vi "jtfa.vi"() -> ()   [LabVIEW 2023]
uses:
  <vilib>/Analysis/4window.llb/windowTd.ctl
  <vilib>/sound2/lvsound2.llb/Sampling Mode.ctl
  <vilib>/sound2/lvsound2.llb/Sound Data Format.ctl
  <vilib>/Analysis/2dsp.llb/Power Spectrum (DBL).vi
  <vilib>/Analysis/4window.llb/Hanning Window (DBL).vi
  <vilib>/Analysis/4window.llb/AllCosWindow (DBL).vi
  <vilib>/sound2/lvsound2.llb/Sound Input Read (DBL).vi
  <vilib>/addons/Time Frequency Analysis/_control.llb/TFA Configure Spectrogram Indicator (Predefined Color Table).vi
  <vilib>/Analysis/NI_AALPro.lvlib
  <vilib>/gmath/NI_Gmath.lvlib
  <vilib>/addons/_Advanced Signal Processing/NI_AdvSigProcTFA.lvlib
  <vilib>/express/express analysis/Spectral/XNode/ExpressSpectralMeasurementsBlockNode.xnode
  <vilib>/express/express analysis/Spectral/Block/exnSpectralBlock spectral measurements RMS poly.vi
  <vilib>/express/express analysis/Spectral/Block/exnSpectralBlock spectral measurements RMS DDT.vi
  <vilib>/Analysis/2dsp.llb/Real FFT.vi
  <vilib>/addons/Time Frequency Analysis/Spectrogram.llb/TFA Online STFT Spectrogram (Waveform).vi
  <vilib>/addons/Time Frequency Analysis/Spectrogram.llb/TFA STFT Spectrogram (Waveform).vi
  <vilib>/addons/Time Frequency Analysis/Transform.llb/TFA STFT (Waveform).vi
panel:
  in  "Num Samples/Ch (N)":dbl(slide)=4096.0 min=1.0 max=48000.0 scale=1.0..4096.0
  in  "Sample Time (s)":dbl(slide)=0.08533333333333333 min=0.01 max=2.0 scale=0.0..2.0
  in  "Frequency Resolution, df (Hz)":dbl(slide)=11.71875 min=1.0 max=24000.0 scale=1.0..100.0
  out "Spectrogram":dbl[][](graph)
  out "phase":dynamicdata(graph)
  out "waveform 2":dynamicdata(graph)
  out "spectrum 2":dynamicdata(graph)
  out "STFT":dbl[][](graph)
  in  "window info":cluster{"type":T1, "length":i32}={"type"=1, "length"=64} {"type" items=["Rectangle"=0, "Hanning"=1, "Hamming"=2, "Blackman-Harris"=3, "Exact Blackman"=4, "Blackman"=5, "Flat Top"=6, "4 Term B-Harris "=7, "7 Term B-Harris"=8, "Low Sidelobe"=9, "Blackman Nuttall"=11, "Triangle"=30, "Bartlett-Hanning"=31, "Bohman"=32, "Parzen"=33, "Welch"=34, "Kaiser"=60, "Dolph-Chebyshev"=61, "Gaussian"=62]}
  in  "time-freq sampling info":cluster{"time steps":i32, "frequency bins":i32}={"time steps"=-1, "frequency bins"=512}
  in  "hanning window":bool
  out "Nyquist Frequency (Hz)":dbl
  in  "stop":bool
  out "waveform":waveform(dbl)(graph)
  out "spectrum":waveform(dbl)(graph)
  # "left off 3am thu 4/11: persisted and got the code to work without errors, added bounds on the inputs to avoid errors (now only if go too low on T manually)\nnext: revisit assignment and what need to get done for that, look at chris sample code"
  # "!! want longer sampling window to get better freq resolution (?)\nb/c freq. res. = 1/time"
  # "w express vi"
  # "- can improve resolution by:\n-- increase length of fft window (but does make time res worse)\n-- increase num bins (increase freq res)"
  # "cut off at -100 dB (y)\ntrim x axis (auto goes\nout to nyq), but only go\nto 15000\n- turn off auto scaling"
  # "not sure why this isn't working but oh well just use chris' in morning"
  # "- our instrument\n- diff notes\n- compare to professional online"
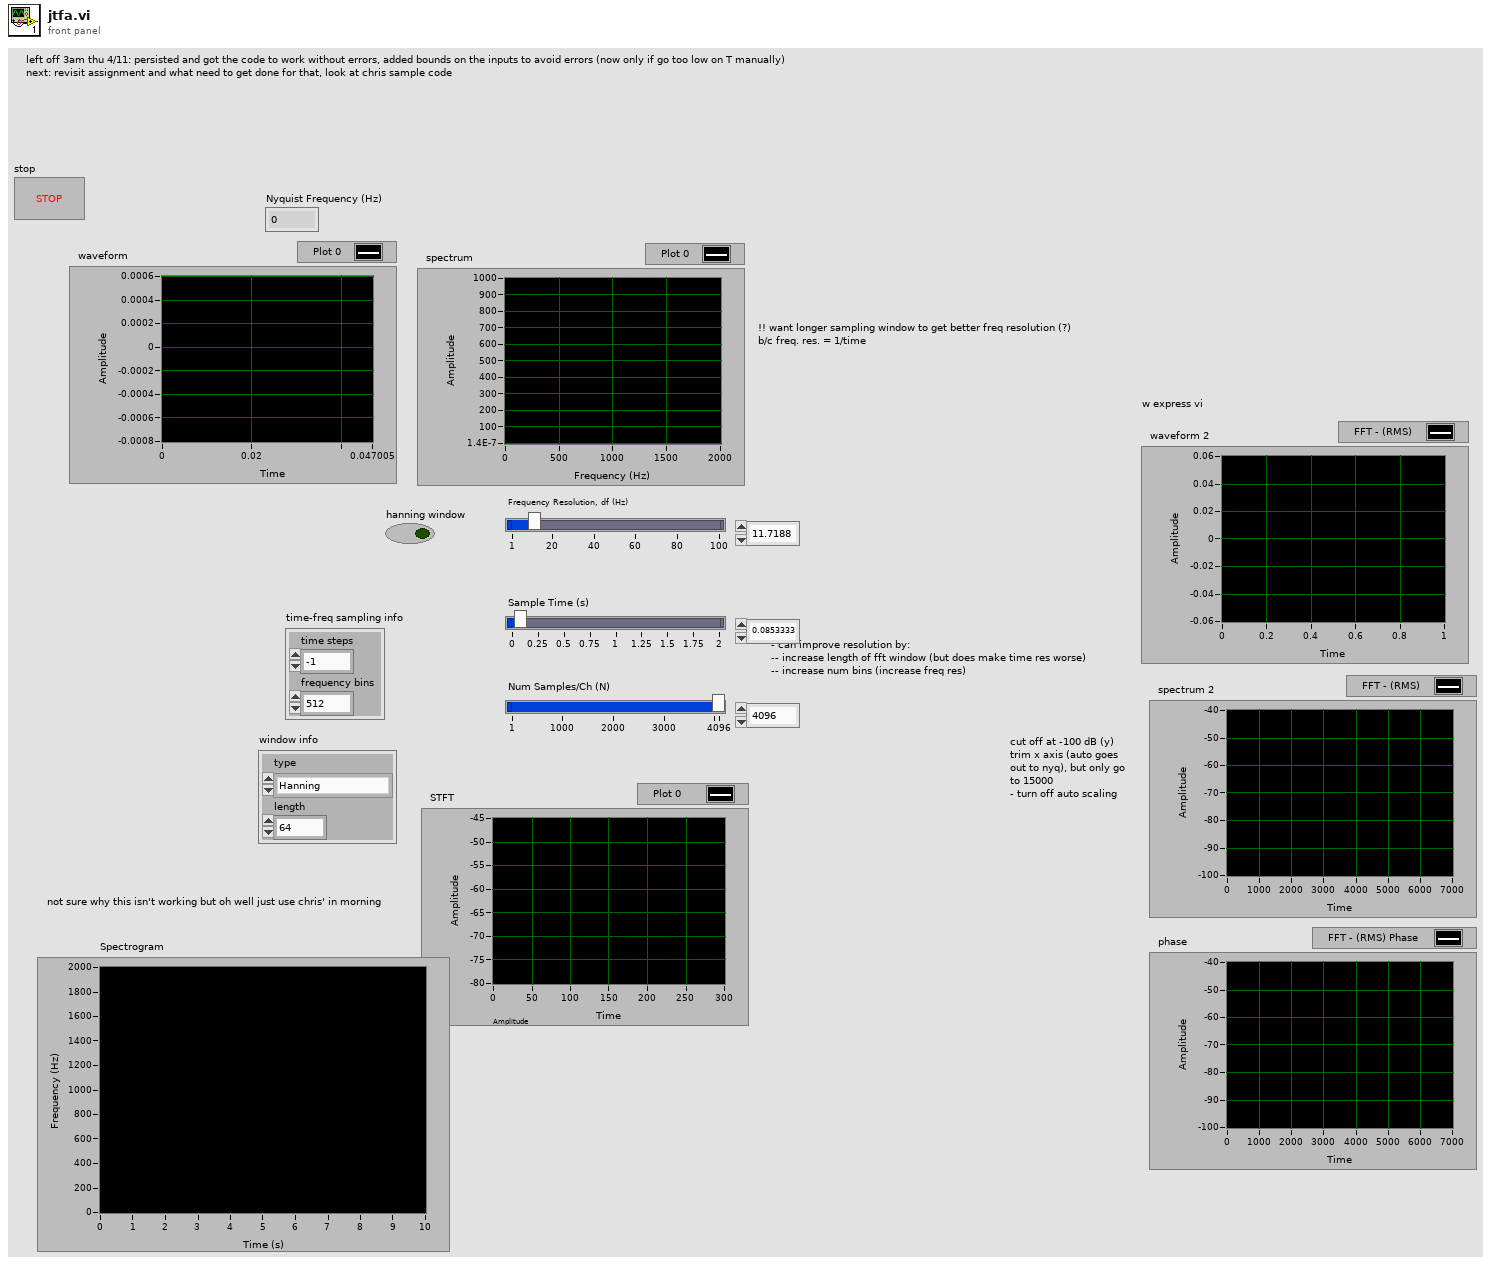
[diagram p1: front panel]
types:
  T1 = typedef "NI_AALPro.lvlib/windowTd.ctl" = u32
  T2 = typedef "Sound Data Format.ctl" = cluster{"sample rate (S/s)":dbl, "number of channels":i32, "bits per sample":i32}
  T3 = typedef "Sampling Mode.ctl" = i32
  T4 = typedef "Sound Input Task ID.ctl" = u32
  T5 = cluster{"averaging mode":u16, "weighting mode":u16, "number of averages":u32}
  T6 = cluster{"dB On (F)":bool, "unwrap phase (F)":bool, "convert to degree (F)":bool}
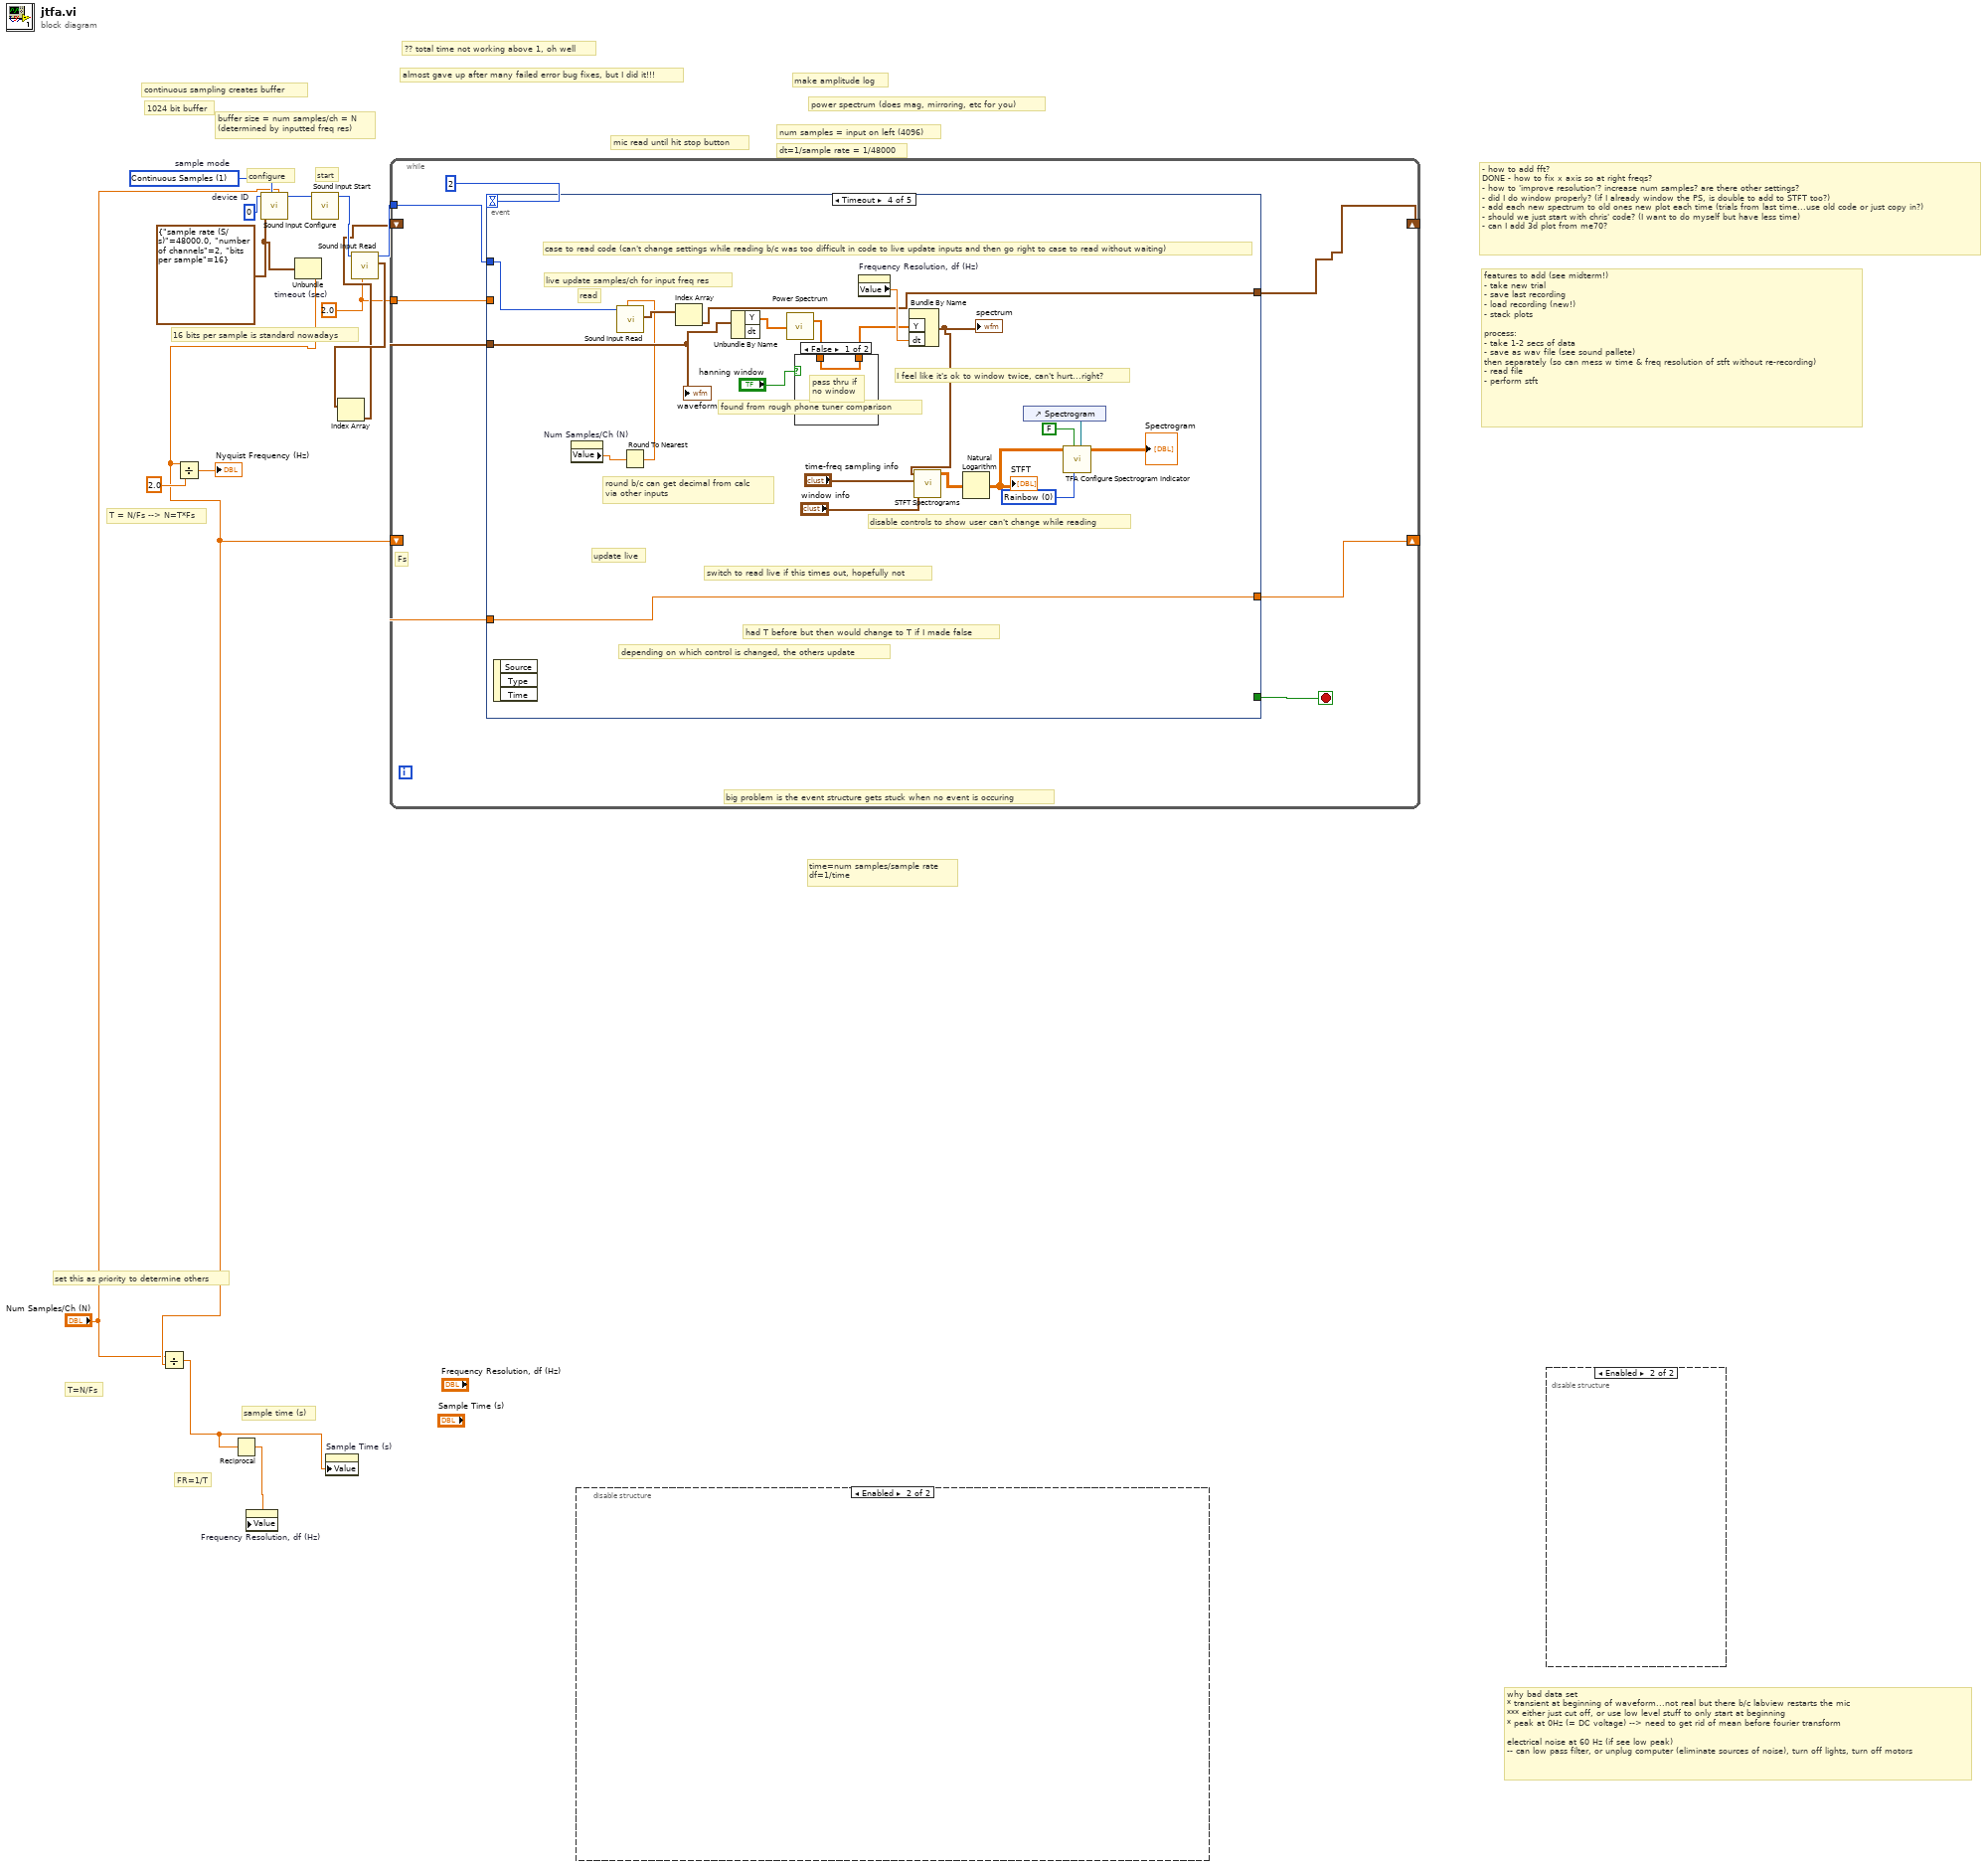
[diagram p0: block diagram]
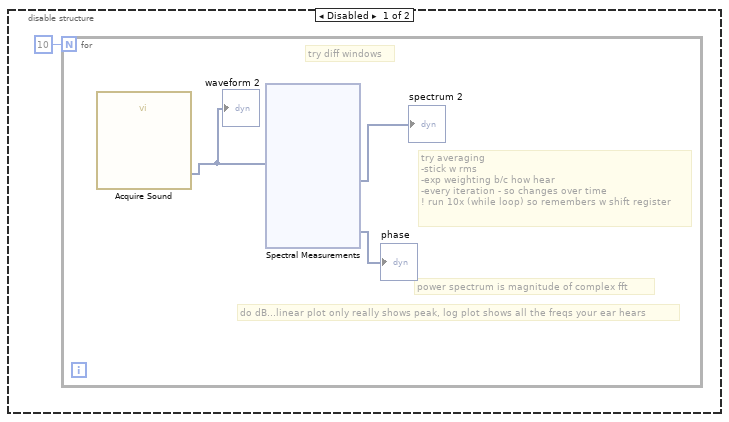
[diagram p2: hidden frame]
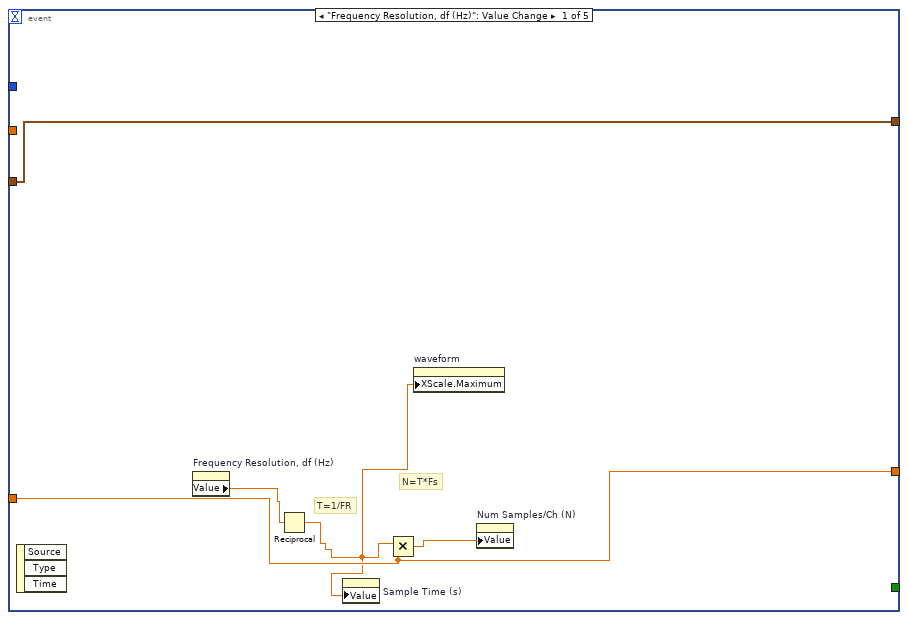
[diagram p3: hidden frame]
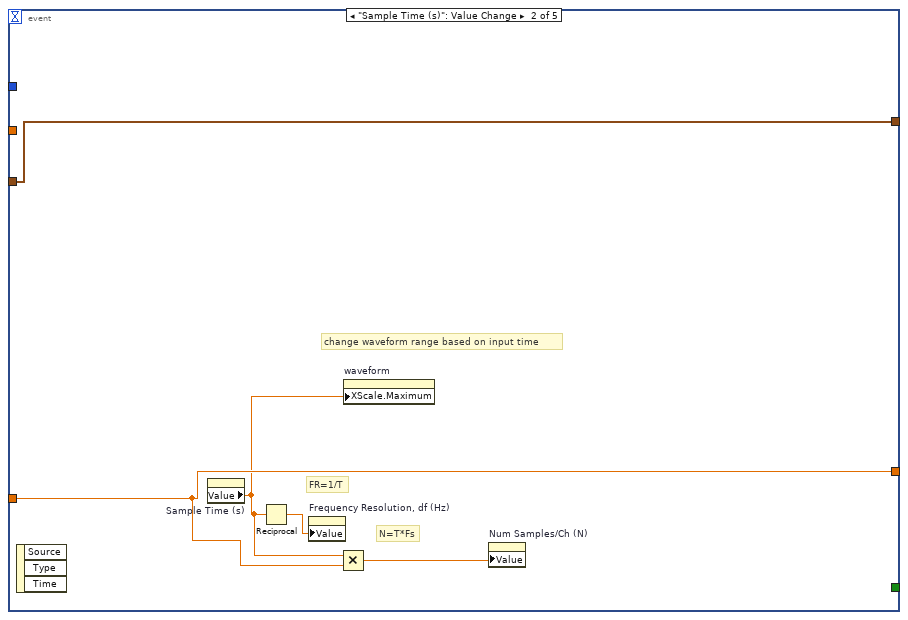
[diagram p4: hidden frame]
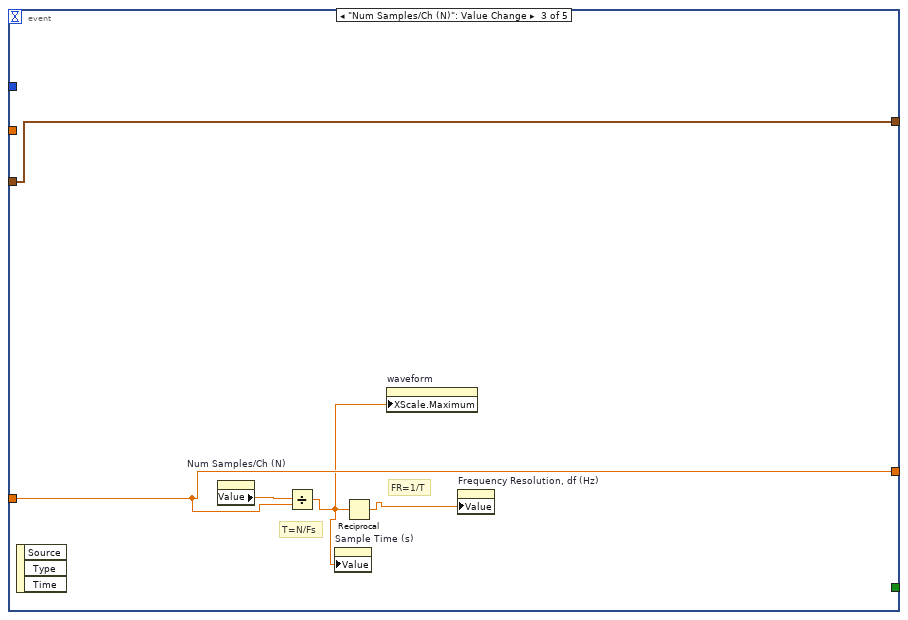
[diagram p5: hidden frame]
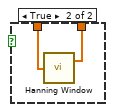
[diagram p6: hidden frame]
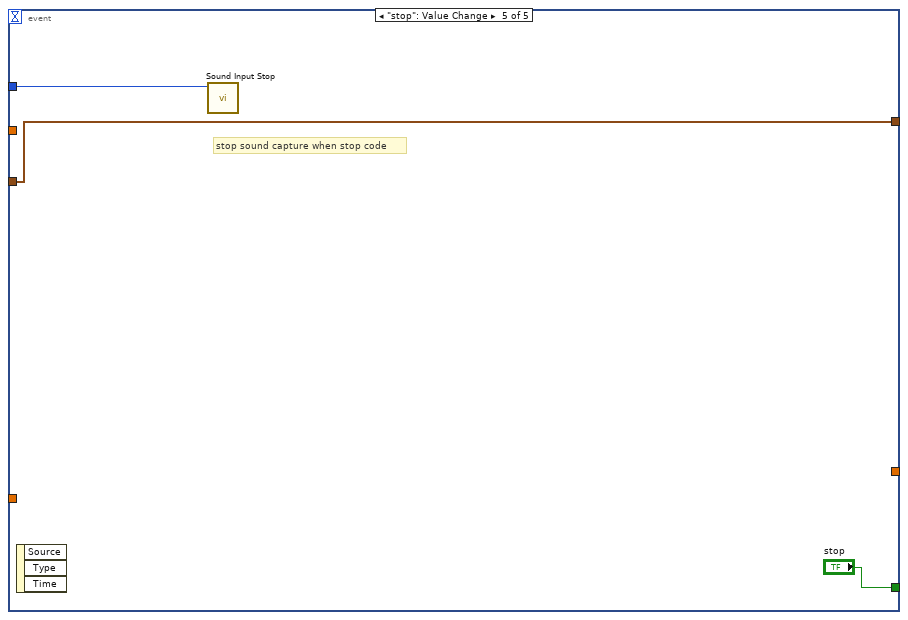
[diagram p7: hidden frame]
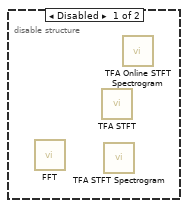
[diagram p8: hidden frame]
diagram:
  w5 = 2.0  # timeout (sec)
  w10 = T2 {"sample rate (S/s)"=48000.0, "number of channels"=2, "bits per sample"=16} ("sound format")
  w14 = u32 0  # device ID
  w15 = T3 1 items=["Finite Samples", "Continuous Samples"]  # sample mode
  # "?? total time not working above 1, oh well"
  # "almost gave up after many failed error bug fixes, but I did it!!!"
  # "FR=1/T"
  # "set this as priority to determine others"
  # "T=N/Fs"
  # "sample time (s)"
  # "T = N/Fs --> N=T*Fs"
  # "time=num samples/sample rate\ndf=1/time"
  # "num samples = input on left (4096)"
  # "dt=1/sample rate = 1/48000"
  # "buffer size = num samples/ch = N\n(determined by inputted freq res)"
  # "start"
  # "configure"
  # "make amplitude log"
  # "power spectrum (does mag, mirroring, etc for you)"
  # "16 bits per sample is standard nowadays"
  # "1024 bit buffer"
  # "continuous sampling creates buffer"
  # "mic read until hit stop button"
  # "why bad data set\n* transient at beginning of waveform...not real but there b/c labview restarts the mic\n*** either just cut off, or use low level stuff to only start at beginning\n* peak at 0Hz (= DC voltage) --> need to get rid of mean before fourier transform\n\nelectrical noise at 60 Hz (if see low peak)\n-- can low pass filter, or unplug computer (eliminate sources of noise), turn off lights, turn off motors"
  # "features to add (see midterm!)\n- take new trial\n- save last recording\n- load recording (new!)\n- stack plots\n\nprocess:\n- take 1-2 secs of data\n- save as wav file (see sound pallete)\nthen separately (so can mess w time & freq resolution of stft without re-recording)\n- read file\n- perform stft"
  # "- how to add fft?\nDONE - how to fix x axis so at right freqs?\n- how to 'improve resolution'? increase num samples? are there other settings?\n- did I do window properly? (if I already window the PS, is double to add to STFT too?)\n- add each new spectrum to old ones new plot each time (trials from last time...use old code or just copy in?)\n- should we just start with chris' code? (I want to do myself but have less time)\n- can I add 3d plot from me70?"
  n1 = call <vilib>:"Sound Input Configure.vi"("number of samples/ch"="Num Samples/Ch (N)", "sample mode"=w15, "sound format"=w10, "device ID"=w14) -> ("task ID"=w13:T4)  [unwired: 6 in, 1 out]
  n2 = Unbundle(w10) -> ("sample rate (S/s)"=w4:dbl)  [unwired: 2 out]
  n3 = Divide(x="Num Samples/Ch (N)", y=w4) -> (x/y=w2:dbl)
  n4 = Divide(x=w4, y=2.0) -> (x/y=→"Nyquist Frequency (Hz)":dbl)
  n5 = Reciprocal(x=w2) -> (1/x=w1:dbl)
  n6 = property on="Frequency Resolution, df (Hz)" class="Slide (strict)"("Value"=w1) -> ()  [unwired: 2 in, 2 out]
  n7 = call <vilib>:"Sound Input Start.vi"("task ID"=w13) -> ("task ID out"=w9:T4)  [unwired: 9 in, 1 out]
  n8 = property on="Sample Time (s)" class="Slide (strict)"("Value"=w2) -> ()  [unwired: 2 in, 2 out]
  n9 = call-poly <vilib>:"Sound Input Read.vi"("timeout (sec)"=w5, "task ID"=w9) -> ("data"=w7:waveform(dbl)[], "task ID out"=w8:T4)  [unwired: 7 in, 1 out]
  n10 = Index Array "Index Array"(array=w7) -> (element=w6:waveform(dbl))  [unwired: 1 in]
  n11 = while {
    shift-right: [w22] -> _
    shift-left: w4 -> [w23]
    tunnel: w8 -> [w20]
    shift-right: [w18] -> _
    shift-left: w6 -> [w17]
    tunnel: w5 -> [w16]
    stop <- w19 stop-if-true
    # "big problem is the event structure gets stuck when no event is occuring"
    # "Fs"
    n12 = event shown="[3] Timeout" {
      selector: _ -> [_ _ _ _ _]
      dyn-events: _ -> [_ _ _ _ _]
      timeout: 2 -> [_ _ _ _ _]
      tunnel: w23 -> [w26 w31 w36 w59 _]
      tunnel: [w26 w31 w36 w59 _] -> w22
      tunnel: w20 -> [_ _ _ w48 w65]
      tunnel: [_ _ _ _ "stop"] -> w19
      tunnel: [w25 w30 w35 w47 w63] -> w18
      tunnel: w17 -> [w25 w30 w35 w46 w63]
      tunnel: w16 -> [_ _ _ _ _]
      event "Frequency Resolution, df (Hz)": Value Change {
        # "N=T*Fs"
        # "T=1/FR"
        n13 = event-data() -> ()  [unwired: 1 in, 3 out]
        n14 = property on="Frequency Resolution, df (Hz)" class="Slide (strict)"() -> ("Value"=w28:dbl)  [unwired: 2 in, 2 out]
        n15 = Reciprocal(x=w28) -> (1/x=w24:dbl)
        n16 = property on="Sample Time (s)" class="Slide (strict)"("Value"=w24) -> ()  [unwired: 2 in, 2 out]
        n17 = Multiply(x=w24, y=w26) -> (x*y=w27:dbl)
        n18 = property on="waveform" class="WFGraph (strict)"("XScale.Maximum"=w24) -> ()  [unwired: 2 in, 2 out]
        n19 = property on="Num Samples/Ch (N)" class="Slide (strict)"("Value"=w27) -> ()  [unwired: 2 in, 2 out]
      }
      event "Sample Time (s)": Value Change {
        # "change waveform range based on input time"
        # "N=T*Fs"
        # "FR=1/T"
        n20 = event-data() -> ()  [unwired: 1 in, 3 out]
        n21 = property on="Sample Time (s)" class="Slide (strict)"() -> ("Value"=w29:dbl)  [unwired: 2 in, 2 out]
        n22 = Reciprocal(x=w29) -> (1/x=w33:dbl)
        n23 = property on="Frequency Resolution, df (Hz)" class="Slide (strict)"("Value"=w33) -> ()  [unwired: 2 in, 2 out]
        n24 = Multiply(x=w29, y=w31) -> (x*y=w32:dbl)
        n25 = property on="waveform" class="WFGraph (strict)"("XScale.Maximum"=w29) -> ()  [unwired: 2 in, 2 out]
        n26 = property on="Num Samples/Ch (N)" class="Slide (strict)"("Value"=w32) -> ()  [unwired: 2 in, 2 out]
      }
      event "Num Samples/Ch (N)": Value Change {
        # "T=N/Fs"
        # "FR=1/T"
        n27 = event-data() -> ()  [unwired: 1 in, 3 out]
        n28 = property on="Num Samples/Ch (N)" class="Slide (strict)"() -> ("Value"=w38:dbl)  [unwired: 2 in, 2 out]
        n29 = Divide(x=w38, y=w36) -> (x/y=w34:dbl)
        n30 = property on="Sample Time (s)" class="Slide (strict)"("Value"=w34) -> ()  [unwired: 2 in, 2 out]
        n31 = Reciprocal(x=w34) -> (1/x=w37:dbl)
        n32 = property on="waveform" class="WFGraph (strict)"("XScale.Maximum"=w34) -> ()  [unwired: 2 in, 2 out]
        n33 = property on="Frequency Resolution, df (Hz)" class="Slide (strict)"("Value"=w37) -> ()  [unwired: 2 in, 2 out]
      }
      event Timeout {
        w40 = u16 0 items=["Rainbow", "Inverse gray", "Gray"] ("color table")
        # "round b/c can get decimal from calc\nvia other inputs"
        # "disable controls to show user can't change while reading"
        # "case to read code (can't change settings while reading b/c was too difficult in code to live update inputs and then go right to case to read without waiting)"
        # "depending on which control is changed, the others update"
        # "live update samples/ch for input freq res"
        # "update live"
        # "I feel like it's ok to window twice, can't hurt...right?"
        # "found from rough phone tuner comparison"
        # "read"
        # "had T before but then would change to T if I made false"
        # "switch to read live if this times out, hopefully not"
        n34 = event-data() -> ()  [unwired: 1 in, 3 out]
        n35 = property on="Num Samples/Ch (N)" class="Slide (strict)"() -> ("Value"=w45:dbl)  [unwired: 2 in, 2 out]
        n36 = Round To Nearest(number=w45) -> (nearest integer value=w44:dbl)
        n37 = call-poly <vilib>:"Sound Input Read.vi"("number of samples/ch"=w44, "task ID"=w48) -> ("data"=w57:waveform(dbl)[])  [unwired: 7 in, 2 out]
        n38 = Index Array "Index Array"(array=w57) -> (element=w47:waveform(dbl))  [unwired: 1 in]
        n39 = Unbundle By Name(w46) -> ("Y"=w56:dbl[])  [unwired: 1 out]
        n40 = call-poly <vilib>:"Power Spectrum.vi"("X"=w56) -> ("Power Spectrum"=w54:dbl[])  [unwired: 1 out]
        n41 = case shown="False" "hanning window" {
          tunnel: w54 -> [w60 w62]
          tunnel: [w60 w61] -> w53
          frame False {
            # "pass thru if\nno window"
          }
          frame True {
            n42 = call-poly <vilib>:"Hanning Window.vi"("X"=w62) -> ("Windowed X"=w61:dbl[])  [unwired: 1 out]
          }
        }
        n43 = property on="Frequency Resolution, df (Hz)" class="Slide (strict)"() -> ("Value"=w58:dbl)  [unwired: 2 in, 2 out]
        n44 = Bundle By Name("Y"=w53, "dt"=w58) -> (w52:waveform(dbl))  [unwired: 1 in]
        "spectrum" <- w52
        n45 = call <vilib>:"STFT Spectrograms.vi"("window info"="window info", "time-freq sampling info"="time-freq sampling info", "X"=w52) -> ("STFT Spectrogram {X}"=w49:dbl[][])  [unwired: 7 in, 1 out]
        n46 = Natural Logarithm(1:w49) -> (0:w41:dbl[][])
        "STFT" <- w41
        n47 = control-ref of="Spectrogram"() -> (w42:refnum<vi>)
        n48 = call-poly <vilib>:"TFA Configure Spectrogram Indicator.vi"("reference of TF spectrogram indicator"=w42, "color table"=w40, "dB on? (F)"=FALSE, "spectrogram"=w41) -> ("TF spectrogram indicator"=→"Spectrogram":dbl[][])  [unwired: 3 in, 4 out]
        "waveform" <- w46
      }
      event "stop": Value Change {
        # "stop sound capture when stop code"
        n49 = event-data() -> ()  [unwired: 1 in, 3 out]
        n50 = call <vilib>:"Sound Input Stop.vi"("task ID"=w65) -> ()  [unwired: 9 in, 2 out]
      }
    }
  }
  n51 = disable-structure shown="Enabled" {
    frame Disabled {
      n52 = for {
        N: 10 -> [_]
        # "do dB...linear plot only really shows peak, log plot shows all the freqs your ear hears"
        # "try diff windows"
        # "power spectrum is magnitude of complex fft"
        # "try averaging\n-stick w rms\n-exp weighting b/c how hear\n-every iteration - so changes over time\n! run 10x (while loop) so remembers w shift register"
        n53 = call "Acquire Sound"() -> ("Data"=w69:dynamicdata)  [unwired: 18 in, 1 out]
        "waveform 2" <- w69
        n54 = xnode "Spectral Measurements"("Signals"=w69) -> ("FFT - (RMS)"=→"spectrum 2":dynamicdata, "Phase"=→"phase":dynamicdata)  [unwired: 2 in, 2 out]
      }
    }
    frame Enabled {
    }
  }
  n55 = disable-structure shown="Enabled" {
    frame Disabled {
      n56 = call-poly <vilib>:"FFT.vi"() -> ()  [unwired: 10 in, 2 out]
      n57 = call-poly <vilib>:"TFA STFT.vi"() -> ()  [unwired: 9 in, 3 out]
      n58 = call-poly <vilib>:"TFA STFT Spectrogram.vi"() -> ()  [unwired: 9 in, 3 out]
      n59 = call-poly <vilib>:"TFA Online STFT Spectrogram.vi"() -> ()  [unwired: 9 in, 3 out]
    }
    frame Enabled {
    }
  }
